vi "Set Property.vi"(8 "error in (no error)":errorcluster, 9 "Value":dbl, 10 "Property":string, 11 "Moving Ripple Noise in":refnum<class "Moving Ripple Noise.lvclass">) -> (0 "error out":errorcluster, 3 "Moving Ripple Noise out":refnum<class "Moving Ripple Noise.lvclass">)   [LabVIEW 2020, in "Moving Ripple Noise.lvclass"]
uses:
  Moving Ripple Noise.lvclass
  Moving Ripple Noise.lvclass/Moving Ripple Noise.ctl
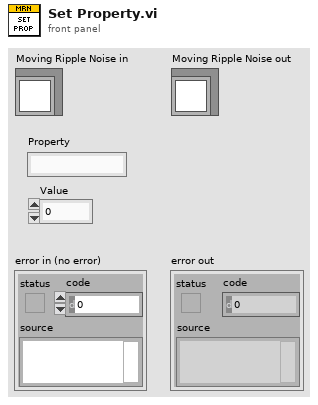
[diagram p1: front panel]
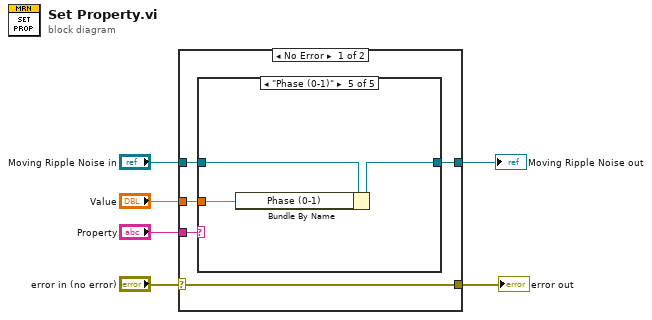
[diagram p0: block diagram]
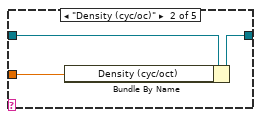
[diagram p3: hidden frame]
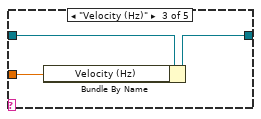
[diagram p4: hidden frame]
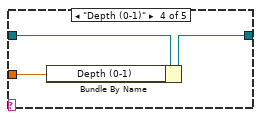
[diagram p5: hidden frame]
diagram:
  n1 = case shown="No Error" "error in (no error)" {
    selector: "error in (no error)" -> [w7 w25]
    tunnel: [w7 w25] -> w4
    tunnel: "Property" -> [w11 _]
    tunnel: "Moving Ripple Noise in" -> [w10 w26]
    tunnel: "Value" -> [w9 _]
    tunnel: [w8 w26] -> w5
    frame No Error {
      n2 = case shown="\"Phase (0-1)\"" w11 {
        tunnel: w10 -> [w12 w15 w18 w21 w24]
        tunnel: w9 -> [_ w14 w17 w20 w23]
        tunnel: [w12 w13 w16 w19 w22] -> w8
        frame "", Default {
        }
        frame "Density (cyc/oc)" {
          n3 = Bundle By Name(cluster=w15, "Density (cyc/oct)"=w14) -> (w13:refnum<class "Moving Ripple Noise.lvclass">)
        }
        frame "Velocity (Hz)" {
          n4 = Bundle By Name(cluster=w18, "Velocity (Hz)"=w17) -> (w16:refnum<class "Moving Ripple Noise.lvclass">)
        }
        frame "Depth (0-1)" {
          n5 = Bundle By Name(cluster=w21, "Depth (0-1)"=w20) -> (w19:refnum<class "Moving Ripple Noise.lvclass">)
        }
        frame "Phase (0-1)" {
          n6 = Bundle By Name(cluster=w24, "Phase (0-1)"=w23) -> (w22:refnum<class "Moving Ripple Noise.lvclass">)
        }
      }
    }
    frame Error {
    }
  }
  "error out" <- w4
  "Moving Ripple Noise out" <- w5
